vi "CircleFinderAI.vi"(6 "Image Name":string="name1", 7 "Session In":T2="cam0", 8 "error in (no error)":errorcluster, 9 "Circle Descriptor":cluster{"Min Radius":dbl, "Max Radius":dbl}={"Min Radius"=50.0, "Max Radius"=80.0}, 10 "Curve Parameters":T7={"Extraction Mode"=0, "Edge Threshold"=100, "Edge Filter Size"=1, "Min Length"=10, "Row Search Step Size"=10, "Col Search Step Size"=100, "Max Endpoint Gap"=100, "Closed"=FALSE, "Subpixel"=FALSE} {"Max Endpoint Gap" min=0; "Col Search Step Size" min=1 max=255 step=1; "Row Search Step Size" min=1 max=255 step=1; "Min Length" min=0; "Edge Filter Size" items=["Fine", "Normal", "Controur Tracing"]; "Edge Threshold" min=1 max=65535 step=1; "Extraction Mode" items=["Normal", "Uniform Regions"]}, 11 "Image Type":T8 items=["Grayscale (U8)", "Grayscale (I16)", "Grayscale (SGL)", "Complex (CSG)", "RGB (U32)", "HSL (U32)", "RGB (U64)", "Grayscale (U16)"]) -> (0 "error out":errorcluster, 1 "AllCircles":T6(array[cluster]) {"Position"."Y" format="%.2f"; "Position"."X" format="%.2f"}, 2 "Circle0":T1, 3 "NumCirclesFound":i32, 5 "Image":T3(plugin-control))   [LabVIEW 2019]
uses:
  <vilib>/vision/Pattern Matching.llb/IMAQ Curve Parameters.ctl
  <vilib>/vision/Shape Detection.llb/ShapeDetectionMatchOptions.ctl
  <vilib>/vision/Pattern Matching.llb/IMAQ Match Range Setting.ctl
  <vilib>/userDefined/High Color/IMAQdx.ctl
  <vilib>/vision/driver/NI_Vision_Acquisition_Software.lvlib
  <vilib>/vision/NI_Vision_Development_Module.lvlib
panel:
  out "Circle0Params":string
  in  "Match Options":T4 {"Range Settings"."Match Constraints" items=["Rotation Angle (degrees)", "Scale Factor (%)", "Occlusion (%)"]}
  # "Range"
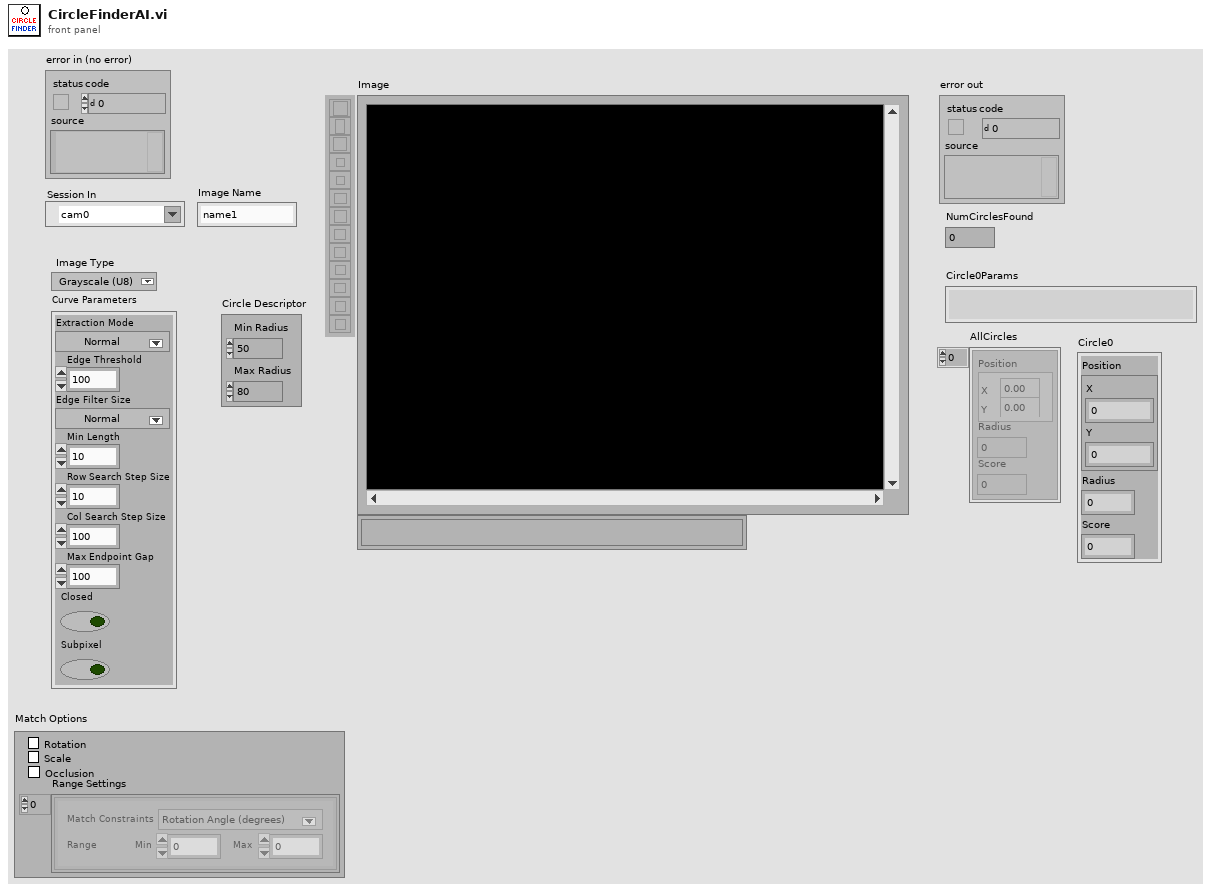
[diagram p1: front panel]
types:
  T1 = cluster{"Position":cluster{"X":sgl, "Y":sgl}, "Radius":dbl, "Score":dbl}
  T2 = typedef "IMAQdx.ctl" = refnum<k21>
  T3 = typedef "IMAQ Image.ctl" = refnum<image>
  T4 = typedef "ShapeDetectionMatchOptions.ctl" = cluster{"Rotation":bool, "Scale":bool, "Occlusion":bool, "Range Settings":T5[]}
  T5 = typedef "IMAQ Match Range Setting.ctl" = cluster{"Match Constraints":u32, "Min":dbl, "Max":dbl}
  T6 = cluster{"Position":cluster{"X":sgl, "Y":sgl}, "Radius":dbl, "Score":dbl}[]
  T7 = typedef "IMAQ Curve Parameters.ctl" = cluster{"Extraction Mode":u32, "Edge Threshold":i32, "Edge Filter Size":u32, "Min Length":i32, "Row Search Step Size":i32, "Col Search Step Size":i32, "Max Endpoint Gap":i32, "Closed":bool, "Subpixel":bool}
  T8 = typedef "Image Type" = u32
  T9 = typedef "IMAQ Circle" = cluster{"Center X":i32, "Center Y":i32, "Inner Radius":i32, "Outer Radius":i32, "Start Angle":dbl, "End Angle":dbl}
  T10 = cluster{"Circles[0]":cluster{"Position":cluster{"X":sgl, "Y":sgl}, "Radius":dbl, "Score":dbl}, "Circles[1]":cluster{"Position":cluster{"X":sgl, "Y":sgl}, "Radius":dbl, "Score":dbl}, "Circles[2]":cluster{"Position":cluster{"X":sgl, "Y":sgl}, "Radius":dbl, "Score":dbl}, "Circles[3]":cluster{"Position":cluster{"X":sgl, "Y":sgl}, "Radius":dbl, "Score":dbl}, "Circles[4]":cluster{"Position":cluster{"X":sgl, "Y":sgl}, "Radius":dbl, "Score":dbl}, "Circles[5]":cluster{"Position":cluster{"X":sgl, "Y":sgl}, "Radius":dbl, "Score":dbl}, "Circles[6]":cluster{"Position":cluster{"X":sgl, "Y":sgl}, "Radius":dbl, "Score":dbl}, "Circles[7]":cluster{"Position":cluster{"X":sgl, "Y":sgl}, "Radius":dbl, "Score":dbl}, "Circles[8]":cluster{"Position":cluster{"X":sgl, "Y":sgl}, "Radius":dbl, "Score":dbl}}
  T11 = typedef "ROI Descriptor" = cluster{"Global Rectangle":i32[], "Contours":cluster{"ID":enum32{"External", "Internal"}, "Type":u32, "Coordinates":i32[]}[]}
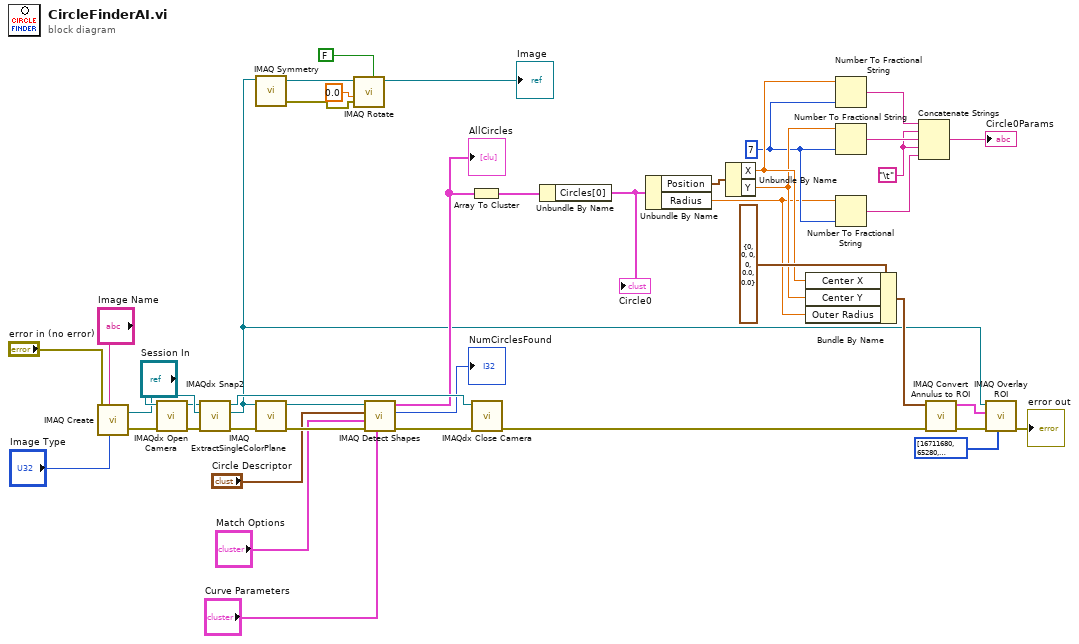
[diagram p0: block diagram]
diagram:
  w6 = "\t"
  w5 = i16 7 ("precision (6)")
  n1 = call "IMAQ Create"("Image Name"="Image Name", "Image Type"="Image Type", "error in (no error)"="error in (no error)") -> ("New Image"=w40:T3, "error out"=w37:errorcluster)  [unwired: 2 in]
  n2 = call <vilib>:"IMAQdx Open Camera.vi"("error in"=w37, "Session In"="Session In") -> ("error out"=w41:errorcluster, "Session Out"=w39:T2)  [unwired: 8 in]
  n3 = call <vilib>:"IMAQdx Snap2.vi"("error in"=w41, "Image In"=w40, "Session In"=w39) -> ("error out"=w33:errorcluster, "Image Out"=w12:T3, "Session Out"=w38:T2)  [unwired: 6 in]
  n4 = call "IMAQ Symmetry"("Image Src"=w12) -> ("error out"=w2:errorcluster, "Image Dst Out"=w16:T3)  [unwired: 4 in]
  n5 = call "IMAQ ExtractSingleColorPlane"("error in (no error)"=w33, "Image Src"=w12) -> ("error out"=w32:errorcluster, "Image Dst Out"=w28:T3)  [unwired: 2 in, 6 out]
  n6 = call "IMAQ Rotate"("Maintain Size"=FALSE, "error in (no error)"=w2, "Angle (degrees)"=sgl 0.0, "Image Src"=w16) -> ("Image Dst Out"=→"Image":T3)  [unwired: 6 in, 1 out]
  n7 = call-poly "IMAQ Detect Shapes"("Curve Parameters"="Curve Parameters", "error in (no error)"=w32, "Match Options"="Match Options", "Circle Descriptor"="Circle Descriptor", "Image"=w28) -> ("error out"=w35:errorcluster, "Number of Matches Returned"=→"NumCirclesFound":i32, "Circles"=w24:T6)  [unwired: 2 in, 2 out]
  "AllCircles" <- w24
  n8 = Array To Cluster(array=w24) -> (cluster=w23:T10)
  n9 = call <vilib>:"IMAQdx Close Camera.vi"("error in"=w35, "Session In"=w38) -> ("error out"=w21:errorcluster)  [unwired: 9 in]
  n10 = Unbundle By Name(w23) -> ("Circles[0]"=w22:T1)
  "Circle0" <- w22
  n11 = Unbundle By Name(w22) -> ("Position"=w25:cluster{"X":sgl, "Y":sgl}, "Radius"=w4:dbl)
  n12 = Unbundle By Name(w25) -> ("X"=w11:sgl, "Y"=w10:sgl)
  n13 = Bundle By Name(cluster=T9 {"Center X"=0, "Center Y"=0, "Inner Radius"=0, "Outer Radius"=0, "Start Angle"=0.0, "End Angle"=0.0} ("Annulus"), "Center X"=w11, "Center Y"=w10, "Outer Radius"=w4) -> (w27:T9)
  n14 = Number To Fractional String(number=w11, precision (6)=w5) -> (F-format string=w9:string)  [unwired: 2 in]
  n15 = Number To Fractional String(number=w10, precision (6)=w5) -> (F-format string=w8:string)  [unwired: 2 in]
  n16 = Number To Fractional String(number=w4, precision (6)=w5) -> (F-format string=w3:string)  [unwired: 2 in]
  n17 = Concatenate Strings(w9, w6, w8, w6, w3) -> (→"Circle0Params":string)
  n18 = call "IMAQ Convert Annulus to ROI"("error in (no error)"=w21, "Annulus"=w27) -> ("error out"=w19:errorcluster, "ROI Descriptor"=w20:T11)  [unwired: 7 in]
  n19 = call "IMAQ Overlay ROI"("Colors (Green)"=u32[] [16711680, 65280, 2626303], "error in (no error)"=w19, "ROI Descriptor"=w20, "Image"=w12) -> ("error out"=→"error out":errorcluster)  [unwired: 6 in, 1 out]
